vi "Group Page.vi"(8 "error in (no error)":errorcluster, 11 "Node Ptr":T1 format="%.0x") -> (0 "error out":errorcluster)   [LabVIEW 2020, in "DSF System Explorer.lvlib"]
uses:
  DSF System Explorer.lvlib
  <vilib>/NI VeriStand/Custom Device API/Custom Device Item Ref.ctl
  DSF Core.lvlibp/Classes/Component User Interface/UI Type.ctl
  <vilib>/NI VeriStand/Custom Device API/Custom Device API.lvlib
  DSF Shared.lvlib
  DSF Core.lvlibp/Classes/Component User Interface/Component User Interfaces.lvclass
  DSF Core.lvlibp/Classes/User Interface/User Interface.lvclass
panel:
  in  "Header":cluster{"Section Name":string}={"Section Name"="Group"}
  in  "Tab Control":enum32{"Settings"}(tab)
  in  "Enable Conversion":bool
  in  "Timeout Behavior":enum8{"Increment Late Count", "Throw Error"}(ring)
  in  "Priority":u64
  in  "Decimation":u64
  in  "Offset":u64
  in  "Direction":enum8{"Tx", "Rx"}(ring)
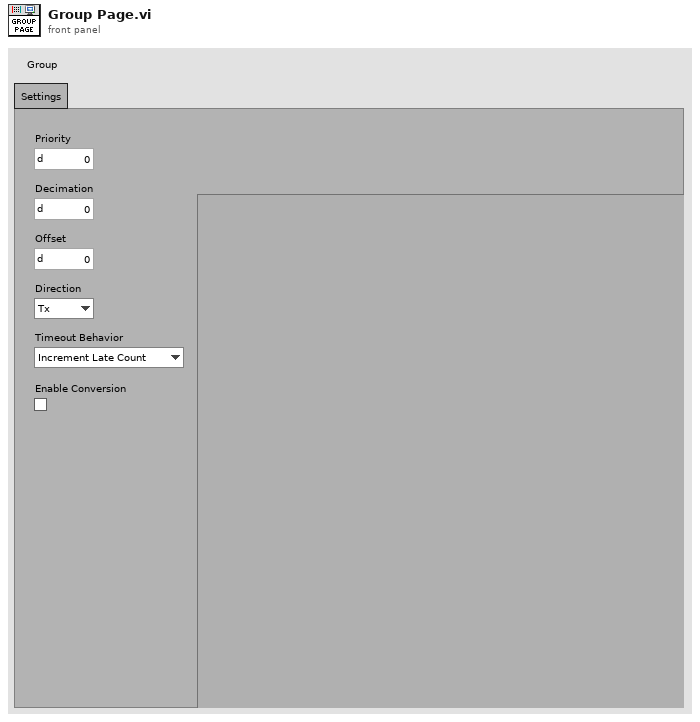
[diagram p1: front panel]
types:
  T1 = typedef "Custom Device API.lvlib/Custom Device Item Ref.ctl" = u64
  T2 = typedef "DSF Core.lvlibp/Component User Interfaces.lvclass/UI Type.ctl" = enum16{"Plugin", "Thread", "Rx Group", "Tx Group", "Rx Transfer", "Tx Transfer", "Rx Channel", "Tx Channel"}
  T3 = typedef "DSF Core.lvlibp/Group Configuration.lvclass/Core Group Configuration.ctl" = cluster{"name":string, "direction":T4, "cycle timing":T5, "timeout behavior":T6, "enable conversion":bool}
  T4 = typedef "DSF Core.lvlibp/DSF Direction.ctl" = enum8{"Tx", "Rx"}
  T5 = typedef "DSF Core.lvlibp/DSF Timing Info.ctl" = cluster{"priority":u64, "decimation":u64, "offset":u64}
  T6 = typedef "DSF Core.lvlibp/DSF Timeout Behavior.ctl" = enum8{"Increment Late Count", "Throw Error"}
  T7 = typedef "DSF Core.lvlibp/User Interface Handler.lvclass/User Interface Ref.ctl" = refnum<vi>
  T8 = typedef "DSF Core.lvlibp/DSF Settings Info.ctl" = cluster{"component":string, "values":cluster{"key":string, "value":string}[]}
  T9 = typedef "Custom Device API.lvlib/Custom Device Commands.ctl" = enum16{"Default", "Item renamed", "Shutdown", "Dynamic button pressed"}
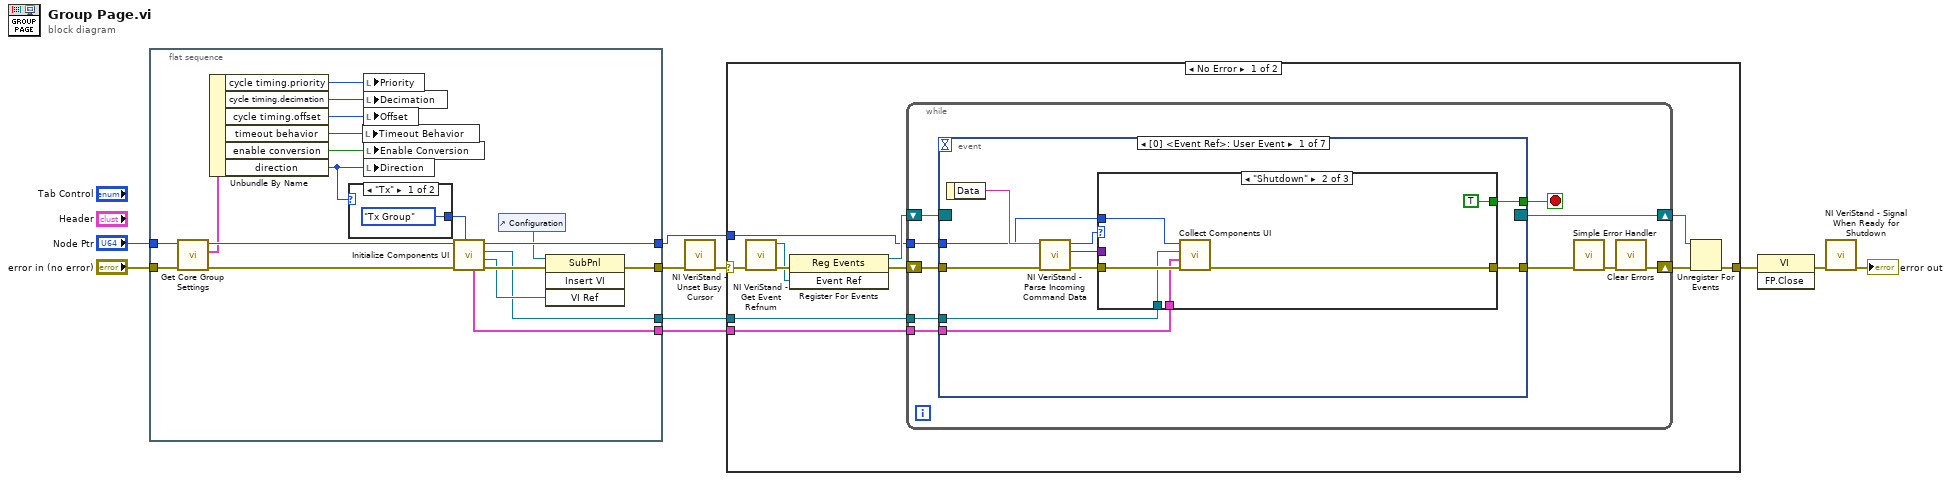
[diagram p0: block diagram]
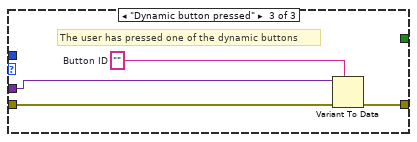
[diagram p3: hidden frame]
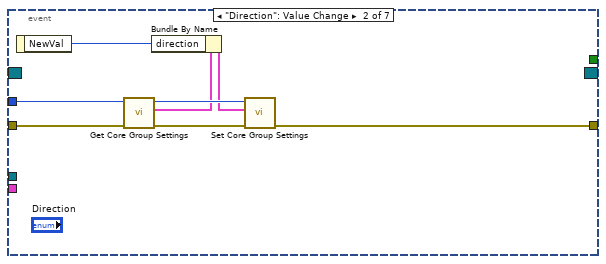
[diagram p4: hidden frame]
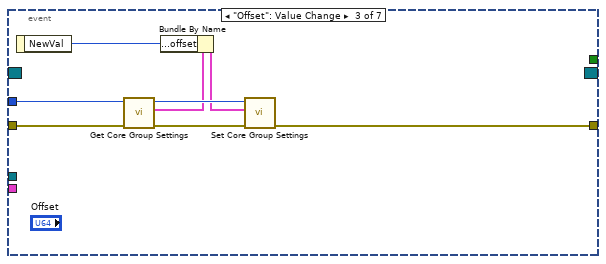
[diagram p5: hidden frame]
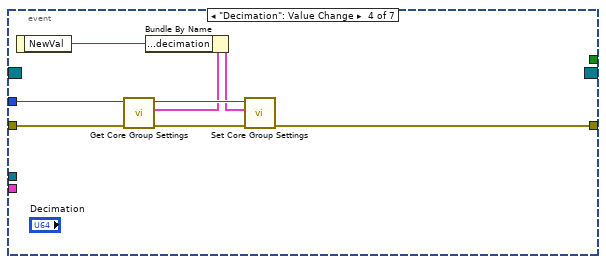
[diagram p6: hidden frame]
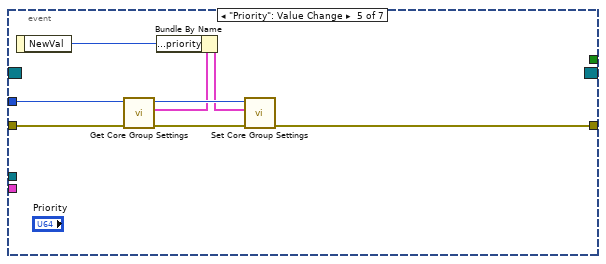
[diagram p7: hidden frame]
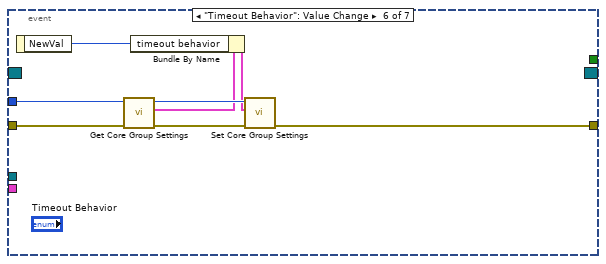
[diagram p8: hidden frame]
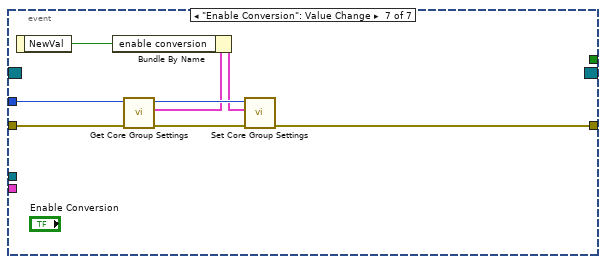
[diagram p9: hidden frame]
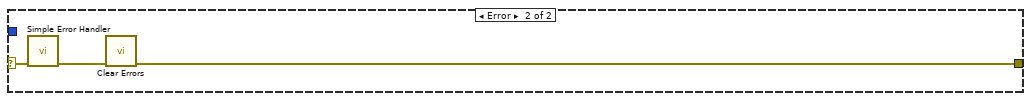
[diagram p10: hidden frame]
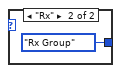
[diagram p11: hidden frame]
diagram:
  n1 = flat-sequence "Initialization code" {
    tunnel: "error in (no error)" -> [w29]
    tunnel: "Node Ptr" -> [w28]
    tunnel: [w19] -> w6
    tunnel: [w17] -> w3
    tunnel: [w18] -> w2
    tunnel: [w11] -> w1
    frame #0 {
      n2 = call "Get Core Group Settings.vi"("error in (no error)"=w29, "Item Ref in"=w28) -> ("error out"=w20:errorcluster, "group configuration"=w15:T3, "Item Ref out"=w16:T1)  [unwired: 7 in]
      n3 = Unbundle By Name(w15) -> ("cycle timing.priority"=w23:u64, "cycle timing.decimation"=w24:u64, "cycle timing.offset"=w25:u64, "timeout behavior"=w26:T6, "enable conversion"=w27:bool, "direction"=w14:T4)
      n4 = case shown="\"Tx\"" w14 {
        tunnel: [UI_Type."Tx Group" ("user interface type") UI_Type."Rx Group" ("user interface type")] -> w13
        frame "Tx" {
        }
        frame "Rx" {
        }
      }
      n5 = local write "Timeout Behavior"(w26) -> ()
      n6 = local write "Priority"(w23) -> ()
      n7 = local write "Decimation"(w24) -> ()
      n8 = local write "Offset"(w25) -> ()
      n9 = local write "Enable Conversion"(w27) -> ()
      n10 = local write "Direction"(w14) -> ()
      n11 = call "Initialize Components UI.vi"("user interface type"=w13, "error in (no error)"=w20, "Item Ref in"=w16) -> ("error out"=w22:errorcluster, "active vi"=w21:T7, "User Interface Handler"=w18:refnum<class "User Interface Handler.lvclass">, "Item Ref out"=w17:T1, "component settings"=w11:T8[])  [unwired: 4 in]
      n12 = control-ref of="Configuration"() -> (w12:refnum<vi>)
      n13 = invoke class="SubPnl" method="Insert VI"(reference=w12, error in=w22, "VI Ref"=w21) -> (error out=w19:errorcluster)  [unwired: 1 in, 3 out]
    }
  }
  n14 = call <vilib>:"NI VeriStand - Unset Busy Cursor.vi"("error in (no error)"=w6) -> ("error out"=w5:errorcluster)  [unwired: 10 out]
  n15 = case shown="No Error" w5 {
    selector: w5 -> [w34 w124]
    tunnel: [w39 w122] -> w10
    tunnel: w3 -> [w35 _]
    tunnel: w2 -> [w33 _]
    tunnel: w1 -> [w32 _]
    frame No Error {
      n16 = call <vilib>:"NI VeriStand - Get Event Refnum.vi"("error in (no error)"=w34) -> ("error out"=w42:errorcluster, "Event Ref"=w38:refnum<user-event>)  [unwired: 9 out]
      n17 = register-events(error in=w42, w38) -> (reference out=w36:refnum<event-registration>, error out=w37:errorcluster)  [unwired: 1 in]
      n18 = while {
        tunnel: w35 -> [w48]
        shift-right: [w45] -> w40
        shift-left: w37 -> [w51]
        shift-right: [w52] -> w41
        shift-left: w36 -> [w50]
        tunnel: w33 -> [w44]
        tunnel: w32 -> [w43]
        stop <- w49 stop-if-true
        n19 = event shown="[0] <Event Ref>: User Event" {
          selector: w50 -> [_ _ _ _ _ _ _]
          dyn-events: [_ _ _ _ _ _ _] -> w52
          timeout: _ -> [_ _ _ _ _ _ _]
          tunnel: w51 -> [w62 w81 w89 w97 w105 w113 w121]
          tunnel: [w58 _ _ _ _ _ _] -> w49
          tunnel: [w57 w77 w85 w93 w101 w109 w117] -> w47
          tunnel: w48 -> [w56 w80 w88 w96 w104 w112 w120]
          tunnel: w44 -> [w54 _ _ _ _ _ _]
          tunnel: w43 -> [w53 _ _ _ _ _ _]
          event User Event {
            n20 = event-data() -> ("Data"=w61:string)  [unwired: 1 out]
            n21 = call <vilib>:"NI VeriStand - Parse Incoming Command Data.vi"("error in (no error)"=w62, "Incoming data"=w61) -> ("error out"=w60:errorcluster, "Outgoing data"=w55:variant, "Action"=w59:T9)  [unwired: 7 out]
            n22 = case shown="\"Shutdown\"" w59 {
              tunnel: w60 -> [w63 w68 w73]
              tunnel: [_ TRUE _] -> w58
              tunnel: [w63 w66 w70] -> w57
              tunnel: w56 -> [_ w67 _]
              tunnel: w55 -> [_ _ w72]
              tunnel: w54 -> [_ w65 _]
              tunnel: w53 -> [_ w64 _]
              frame "Default", Default {
              }
              frame "Shutdown" {
                n23 = call "Collect Components UI.vi"("error in (no error)"=w68, "current component settings"=w64, "User Interface Handler"=w65, "Item Ref in"=w67) -> ("error out"=w66:errorcluster)  [unwired: 6 in, 1 out]
              }
              frame "Dynamic button pressed" {
                w71 = ""  # Button ID
                # "The user has pressed one of the dynamic buttons"
                n24 = Variant To Data(error in=w73, type=w71, Variant=w72) -> (error out=w70:errorcluster)  [unwired: 1 out]
              }
            }
          }
          event "Direction": Value Change {
            n25 = event-data() -> ("NewVal"=w76:enum8{"Tx", "Rx"})  [unwired: 1 out]
            n26 = call "Get Core Group Settings.vi"("error in (no error)"=w81, "Item Ref in"=w80) -> ("error out"=w79:errorcluster, "group configuration"=w75:T3, "Item Ref out"=w78:T1)  [unwired: 7 in]
            n27 = Bundle By Name(cluster=w75, "direction"=w76) -> (w74:T3)
            n28 = call "Set Core Group Settings.vi"("error in (no error)"=w79, "group configuration"=w74, "Item Ref in"=w78) -> ("error out"=w77:errorcluster)  [unwired: 7 in, 1 out]
          }
          event "Offset": Value Change {
            n29 = event-data() -> ("NewVal"=w84:u64)  [unwired: 1 out]
            n30 = call "Get Core Group Settings.vi"("error in (no error)"=w89, "Item Ref in"=w88) -> ("error out"=w87:errorcluster, "group configuration"=w83:T3, "Item Ref out"=w86:T1)  [unwired: 7 in]
            n31 = Bundle By Name(cluster=w83, "cycle timing.offset"=w84) -> (w82:T3)
            n32 = call "Set Core Group Settings.vi"("error in (no error)"=w87, "group configuration"=w82, "Item Ref in"=w86) -> ("error out"=w85:errorcluster)  [unwired: 7 in, 1 out]
          }
          event "Decimation": Value Change {
            n33 = event-data() -> ("NewVal"=w92:u64)  [unwired: 1 out]
            n34 = call "Get Core Group Settings.vi"("error in (no error)"=w97, "Item Ref in"=w96) -> ("error out"=w95:errorcluster, "group configuration"=w91:T3, "Item Ref out"=w94:T1)  [unwired: 7 in]
            n35 = Bundle By Name(cluster=w91, "cycle timing.decimation"=w92) -> (w90:T3)
            n36 = call "Set Core Group Settings.vi"("error in (no error)"=w95, "group configuration"=w90, "Item Ref in"=w94) -> ("error out"=w93:errorcluster)  [unwired: 7 in, 1 out]
          }
          event "Priority": Value Change {
            n37 = event-data() -> ("NewVal"=w100:u64)  [unwired: 1 out]
            n38 = call "Get Core Group Settings.vi"("error in (no error)"=w105, "Item Ref in"=w104) -> ("error out"=w103:errorcluster, "group configuration"=w99:T3, "Item Ref out"=w102:T1)  [unwired: 7 in]
            n39 = Bundle By Name(cluster=w99, "cycle timing.priority"=w100) -> (w98:T3)
            n40 = call "Set Core Group Settings.vi"("error in (no error)"=w103, "group configuration"=w98, "Item Ref in"=w102) -> ("error out"=w101:errorcluster)  [unwired: 7 in, 1 out]
          }
          event "Timeout Behavior": Value Change {
            n41 = event-data() -> ("NewVal"=w108:enum8{"Increment Late Count", "Throw Error"})  [unwired: 1 out]
            n42 = call "Get Core Group Settings.vi"("error in (no error)"=w113, "Item Ref in"=w112) -> ("error out"=w111:errorcluster, "group configuration"=w107:T3, "Item Ref out"=w110:T1)  [unwired: 7 in]
            n43 = Bundle By Name(cluster=w107, "timeout behavior"=w108) -> (w106:T3)
            n44 = call "Set Core Group Settings.vi"("error in (no error)"=w111, "group configuration"=w106, "Item Ref in"=w110) -> ("error out"=w109:errorcluster)  [unwired: 7 in, 1 out]
          }
          event "Enable Conversion": Value Change {
            n45 = event-data() -> ("NewVal"=w116:bool)  [unwired: 1 out]
            n46 = call "Get Core Group Settings.vi"("error in (no error)"=w121, "Item Ref in"=w120) -> ("error out"=w119:errorcluster, "group configuration"=w115:T3, "Item Ref out"=w118:T1)  [unwired: 7 in]
            n47 = Bundle By Name(cluster=w115, "enable conversion"=w116) -> (w114:T3)
            n48 = call "Set Core Group Settings.vi"("error in (no error)"=w119, "group configuration"=w114, "Item Ref in"=w118) -> ("error out"=w117:errorcluster)  [unwired: 7 in, 1 out]
          }
        }
        n49 = call <vilib>:"Simple Error Handler.vi"("error in (no error)"=w47) -> ("error out"=w46:errorcluster)  [unwired: 1 in, 7 out]
        n50 = call <vilib>:"Clear Errors.vi"("error in (no error)"=w46) -> ("error out"=w45:errorcluster)  [unwired: 1 in, 5 out]
      }
      n51 = Unregister For Events(event registration refnum=w41, error in=w40) -> (error out=w39:errorcluster)
    }
    frame Error {
      n52 = call <vilib>:"Simple Error Handler.vi"("error in (no error)"=w124) -> ("error out"=w123:errorcluster)  [unwired: 1 in, 7 out]
      n53 = call <vilib>:"Clear Errors.vi"("error in (no error)"=w123) -> ("error out"=w122:errorcluster)  [unwired: 1 in, 5 out]
    }
  }
  n54 = invoke class="VI" method="FP.Close"(error in=w10) -> (error out=w9:errorcluster)  [unwired: 2 in, 2 out]
  n55 = call <vilib>:"NI VeriStand - Signal When Ready for Shutdown.vi"("error in (no error)"=w9) -> ("error out"=→"error out":errorcluster)  [unwired: 10 out]
